vi "Main UI.vi"(8 "error in (no error)":errorcluster, 11 "TouchControl in":refnum<class "TouchControl.lvclass">) -> (0 "error out":errorcluster, 3 "TouchControl out":refnum<class "TouchControl.lvclass">)   [LabVIEW 2022 SP3, in "TouchControl.lvlib" / "TouchControl.lvclass"]
uses:
  TouchControl.lvclass
  <vilib>/IlluminatedG/IG OOPanel/OOPanel/Manager/Manager.lvclass
  MuxPanel/MuxPanel.lvclass
  LightsPanel/LightsPanel.lvclass
  AudioMonPanel/AudioMonPanel.lvclass
  TouchControl.lvclass/TouchControl.ctl
  <vilib>/IlluminatedG/IG OOPanel/OOPanel/Panel/Panel.lvclass
  TouchControl.lvlib
panel:
  in  "10":bool
  in  "9":bool
  in  "8":bool
  in  "7":bool
  in  "6":bool
  in  "5":bool
  in  "4":bool
  in  "3":bool
  in  "2":bool
  in  "1":bool
  in  "Close":bool
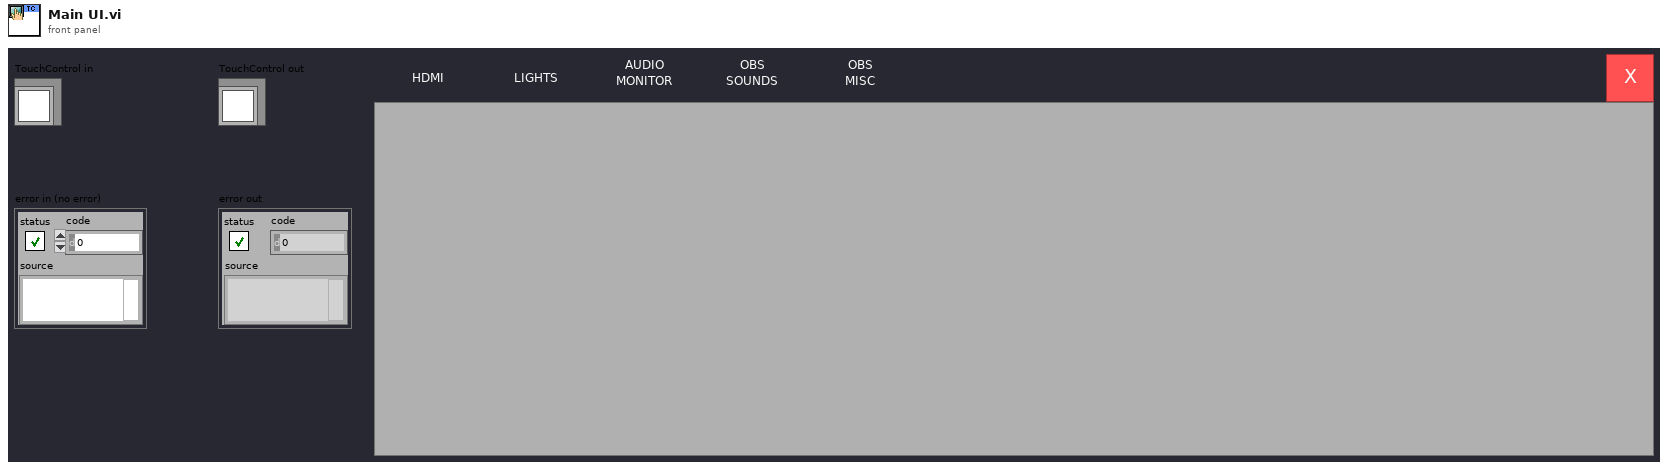
[diagram p1: front panel]
types:
  T1 = enum32{"Invalid", "Standard", "Closed", "Hidden", "Minimized", "Maximized"}
  T2 = enum8{"Enabled", "Disabled", "Disabled and Grayed Out"}
  T3 = enum32{"invalid app kind", "Development System", "Run Time System", "Student Edition", "Embedded LabVIEW", "Evaluation", "Custom"}
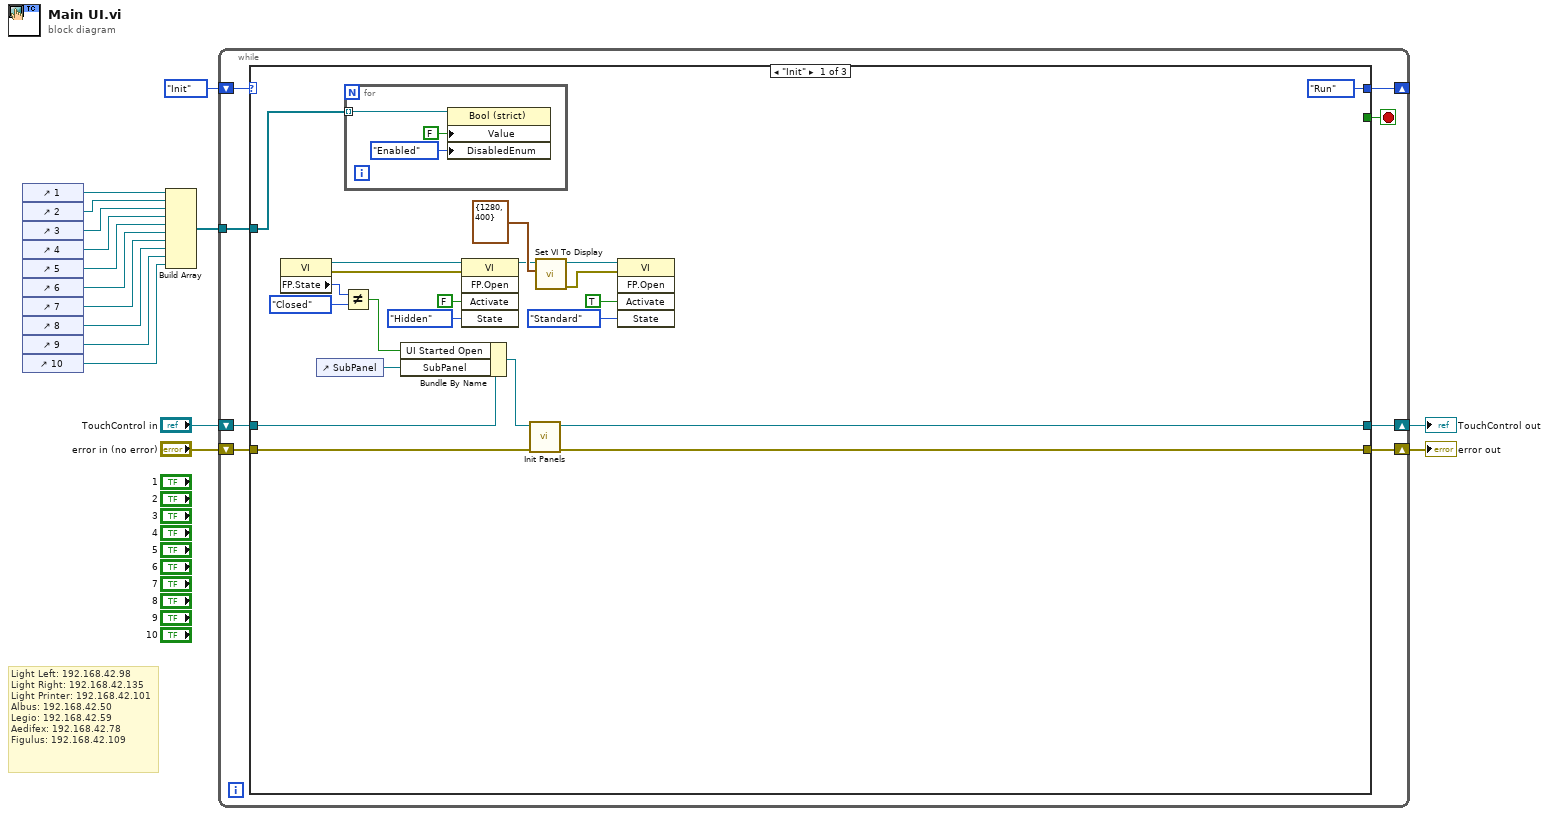
[diagram p0: block diagram]
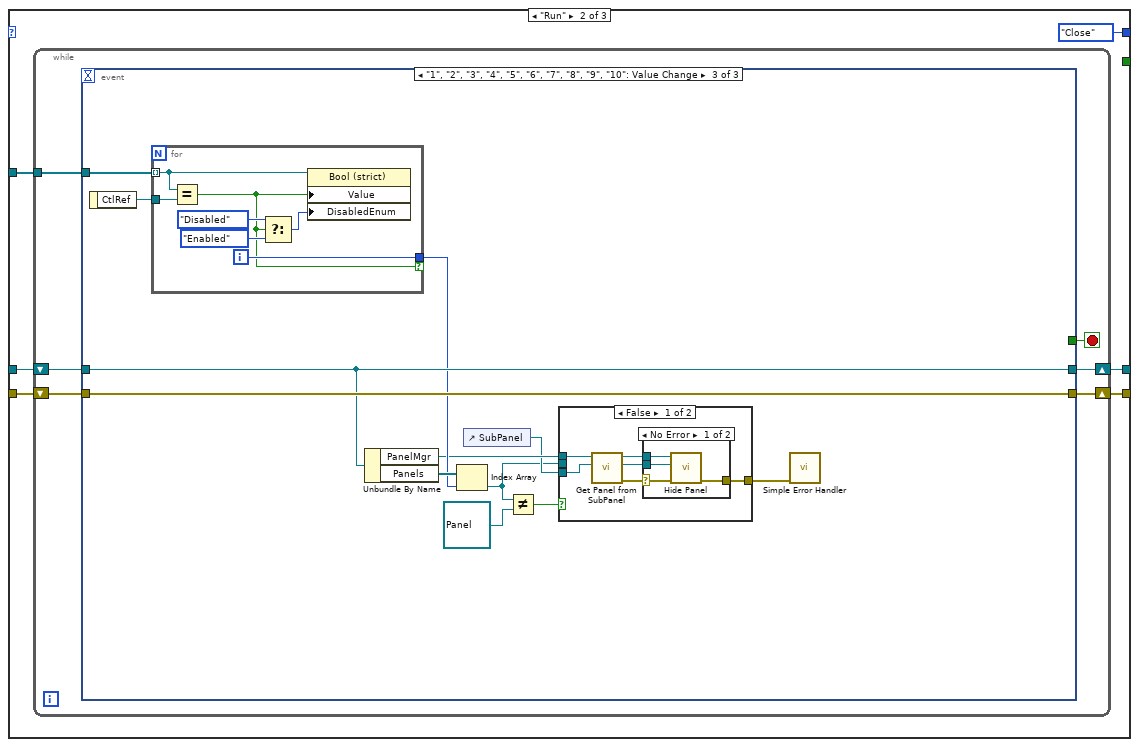
[diagram p2: hidden frame]
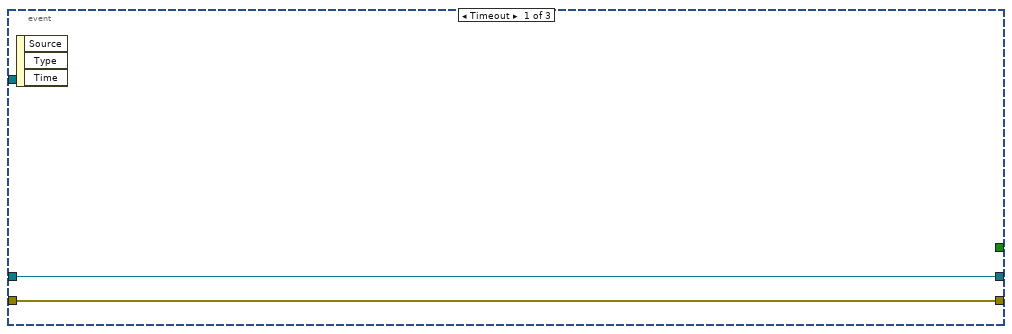
[diagram p3: hidden frame]
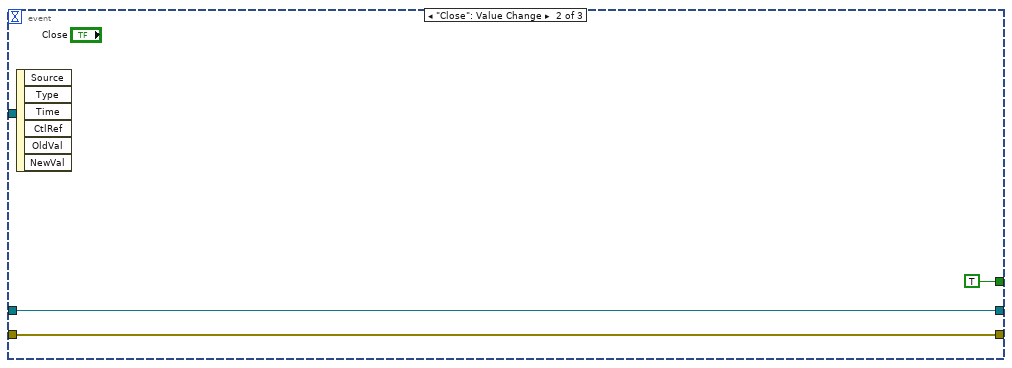
[diagram p4: hidden frame]
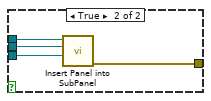
[diagram p6: hidden frame]
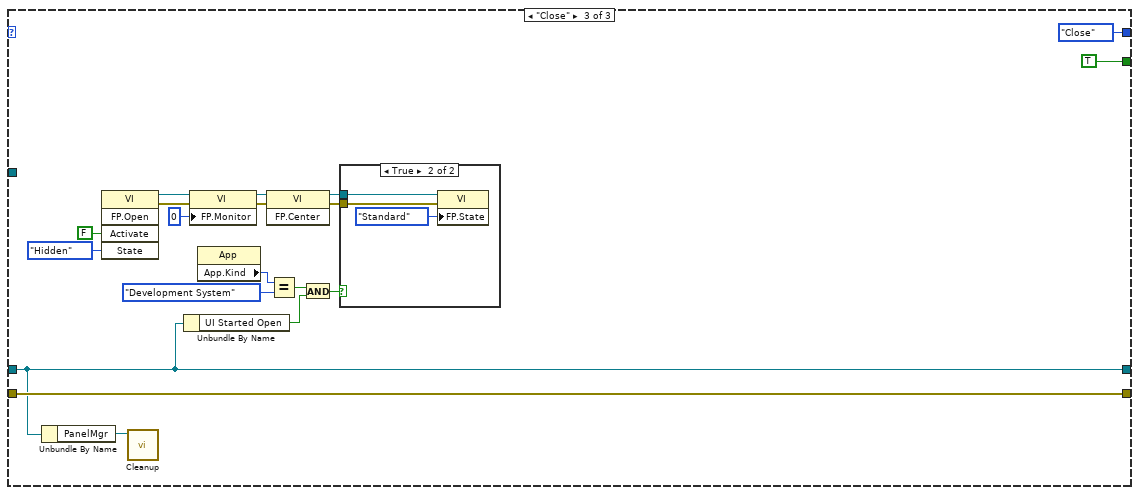
[diagram p7: hidden frame]
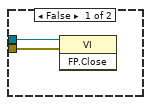
[diagram p8: hidden frame]
diagram:
  # "Light Left: 192.168.42.98\nLight Right: 192.168.42.135\nLight Printer: 192.168.42.101\nAlbus: 192.168.42.50\nLegio: 192.168.42.59\nAedifex: 192.168.42.78\nFigulus: 192.168.42.109"
  n1 = control-ref of="1"() -> (w11:refnum<vi>)
  n2 = control-ref of="2"() -> (w10:refnum<vi>)
  n3 = control-ref of="3"() -> (w9:refnum<vi>)
  n4 = control-ref of="4"() -> (w8:refnum<vi>)
  n5 = control-ref of="5"() -> (w7:refnum<vi>)
  n6 = control-ref of="6"() -> (w6:refnum<vi>)
  n7 = control-ref of="7"() -> (w5:refnum<vi>)
  n8 = control-ref of="8"() -> (w4:refnum<vi>)
  n9 = control-ref of="9"() -> (w3:refnum<vi>)
  n10 = control-ref of="10"() -> (w2:refnum<vi>)
  n11 = Build Array(w11, w10, w9, w8, w7, w6, w5, w4, w3, w2) -> (w1:refnum<vi>[])
  n12 = while {
    shift-right: [w23] -> _
    shift-left: enum16{"Init", "Run", "Close"}."Init" -> [w24]
    shift-right: [w19] -> w13
    shift-left: "TouchControl in" -> [w21]
    shift-right: [w18] -> w12
    shift-left: "error in (no error)" -> [w20]
    tunnel: w1 -> [w17]
    stop <- w22 stop-if-true
    n13 = case shown="\"Init\"" w24 {
      tunnel: [enum16{"Init", "Run", "Close"}."Run" enum16{"Init", "Run", "Close"}."Close" enum16{"Init", "Run", "Close"}."Close"] -> w23
      tunnel: [_ _ TRUE] -> w22
      tunnel: w21 -> [w30 w53 w100]
      tunnel: w20 -> [w44 w52 w115]
      tunnel: [w26 w51 w100] -> w19
      tunnel: [w28 w50 w115] -> w18
      tunnel: w17 -> [w25 w49 _]
      frame "Init" {
        n14 = property class="VI"() -> (reference out=w34:refnum<vi>, error out=w35:errorcluster, "FP.State"=w33:T1)  [unwired: 2 in]
        n15 = control-ref of="SubPanel"() -> (w29:refnum<vi>)
        n16 = Not Equal?(x=w33, y=T1."Closed") -> (x != y?=w31:bool)
        n17 = for {
          tunnel: w25 -> [w48] mode=indexing
          n18 = property class="Bool (strict)"(reference=w48, "Value"=FALSE, "DisabledEnum"=T2."Enabled" ("Disabled")) -> ()  [unwired: 1 in, 2 out]
        }
        n19 = Bundle By Name(cluster=w30, "UI Started Open"=w31, "SubPanel"=w29) -> (w27:refnum<class "TouchControl.lvclass">)
        n20 = invoke class="VI" method="FP.Open"(reference=w34, error in=w35, "Activate"=FALSE ("Activate?"), "State"=T1."Hidden") -> (reference out=w40:refnum<vi>)  [unwired: 1 in, 4 out]
        n21 = call "Init Panels.vi"("error in (no error)"=w44, "TouchControl in"=w27) -> ("error out"=w28:errorcluster, "TouchControl out"=w26:refnum<class "TouchControl.lvclass">)  [unwired: 8 in]
        n22 = call "Set VI To Display.vi"("Display Size"=cluster{"Width":i16, "Height":i16} {"Width"=1280, "Height"=400}, "VI In"=w40) -> ("error out"=w36:errorcluster, "VI"=w39:refnum<vi>)  [unwired: 7 in, 1 out]
        n23 = invoke class="VI" method="FP.Open"(reference=w39, error in=w36, "Activate"=TRUE ("Activate?"), "State"=T1."Standard") -> ()  [unwired: 1 in, 5 out]
      }
      frame "Run" {
        n24 = while {
          shift-right: [w58] -> w51
          shift-left: w53 -> [w60]
          shift-right: [w57] -> w50
          shift-left: w52 -> [w59]
          tunnel: w49 -> [w55]
          stop <- w56 stop-if-true
          n25 = event shown="[2] \"1\", \"2\", \"3\", \"4\", \"5\", \"6\", \"7\", \"8\", \"9\", \"10\": Value Change" {
            selector: _ -> [_ _ _]
            dyn-events: _ -> [_ _ _]
            timeout: _ -> [_ _ _]
            tunnel: w60 -> [w62 w65 w74]
            tunnel: w59 -> [w61 w64 w77]
            tunnel: [w62 w65 w74] -> w58
            tunnel: [w61 w64 w77] -> w57
            tunnel: [_ TRUE _] -> w56
            tunnel: w55 -> [_ _ w76]
            event Timeout {
              n26 = event-data() -> ()  [unwired: 1 in, 3 out]
            }
            event "Close": Value Change {
              n27 = event-data() -> ()  [unwired: 1 in, 6 out]
            }
            event "1", "2", "3", "4", "5", "6", "7", "8", "9", "10": Value Change {
              n28 = event-data() -> ("CtlRef"=w75:refnum<vi>)  [unwired: 1 in]
              n29 = for {
                tunnel: w76 -> [w98] mode=indexing
                tunnel: w75 -> [w97]
                tunnel: [w93] -> w72 if=w92
                i -> [w93]
                n30 = Equal?(x=w98, y=w97) -> (x = y?=w92:bool)
                n31 = Select(t=T2."Disabled" ("Disabled"), s=w92, f=T2."Enabled" ("Disabled")) -> (s? t:f=w94:T2)
                n32 = property class="Bool (strict)"(reference=w98, "Value"=w92, "DisabledEnum"=w94) -> ()  [unwired: 1 in, 2 out]
              }
              n33 = Unbundle By Name(w74) -> ("PanelMgr"=w71:refnum<class "Manager.lvclass">, "Panels"=w73:refnum<class "Panel.lvclass">[])
              n34 = Index Array(array=w73, index=w72) -> (element=w68:refnum<class "Panel.lvclass">)
              n35 = control-ref of="SubPanel"() -> (w70:refnum<vi>)
              n36 = Not Equal?(x=w68, y=refnum<class "Panel.lvclass"> refnum) -> (x != y?=w66:bool)
              n37 = case shown="False" w66 {
                tunnel: w71 -> [w83 w91]
                tunnel: w70 -> [w82 w90]
                tunnel: [w78 w89] -> w69
                tunnel: w68 -> [_ w88]
                frame False {
                  n38 = call <vilib>:"Get Panel from SubPanel.vi"("SubPanel"=w82, "Manager in"=w83) -> ("error out"=w79:errorcluster, "Panel"=w80:refnum<class "Panel.lvclass">, "Manager out"=w81:refnum<class "Manager.lvclass">)  [unwired: 6 in, 1 out]
                  n39 = case shown="No Error" w79 {
                    selector: w79 -> [w85 _]
                    tunnel: w81 -> [w87 _]
                    tunnel: w80 -> [w86 _]
                    tunnel: [w84 _] -> w78
                    frame No Error {
                      n40 = call <vilib>:"Hide Panel.vi"("error in (no error)"=w85, "Panel In"=w86, "Manager in"=w87) -> ("error out"=w84:errorcluster)  [unwired: 6 in, 2 out]
                    }
                    frame Error {
                    }
                  }
                }
                frame True {
                  n41 = call <vilib>:"Insert Panel into SubPanel.vi"("SubPanel"=w90, "Panel In"=w88, "Manager in"=w91) -> ("error out"=w89:errorcluster)  [unwired: 6 in, 2 out]
                }
              }
              n42 = call <vilib>:"Simple Error Handler.vi"("error in (no error)"=w69) -> ()  [unwired: 4 in, 5 out]
            }
          }
        }
      }
      frame "Close" {
        n43 = Unbundle By Name(w100) -> ("PanelMgr"=w99:refnum<class "Manager.lvclass">)
        n44 = invoke class="VI" method="FP.Open"("Activate"=FALSE ("Activate?"), "State"=T1."Hidden") -> (reference out=w112:refnum<vi>, error out=w108:errorcluster)  [unwired: 3 in, 3 out]
        n45 = call <vilib>:"Cleanup.vi"("Manager in"=w99) -> ()  [unwired: 8 in, 3 out]
        n46 = Unbundle By Name(w100) -> ("UI Started Open"=w102:bool)
        n47 = property class="VI"(reference=w112, error in=w108, "FP.Monitor"=u16 0 ("Front Panel Window:Monitor")) -> (reference out=w110:refnum<vi>, error out=w109:errorcluster)
        n48 = property class="App"() -> ("App.Kind"=w105:T3)  [unwired: 2 in, 2 out]
        n49 = invoke class="VI" method="FP.Center"(reference=w110, error in=w109) -> (reference out=w106:refnum<vi>, error out=w107:errorcluster)  [unwired: 1 in, 1 out]
        n50 = Equal?(x=w105, y=T3."Development System") -> (x = y?=w103:bool)
        n51 = And(x=w103, y=w102) -> (x .and. y?=w101:bool)
        n52 = case shown="True" w101 {
          tunnel: w107 -> [w118 w121]
          tunnel: w106 -> [w119 w122]
          frame False {
            n53 = invoke class="VI" method="FP.Close"(reference=w119, error in=w118) -> ()  [unwired: 1 in, 3 out]
          }
          frame True {
            n54 = property class="VI"(reference=w122, error in=w121, "FP.State"=T1."Standard" ("Front Panel Window:State")) -> ()  [unwired: 2 out]
          }
        }
      }
    }
  }
  "error out" <- w12
  "TouchControl out" <- w13
